vi "Determine Transmission.vi"(6 "Channel Value Change":bool, 8 "Detect?":bool[](array[boolean]), 9 "Values":dbl[](array[numeric]), 10 "Trigger VS Index":i32, 11 "Transmit Trigger":T1) -> (3 "Transmit":bool)   [LabVIEW 2015, in "Protection and Rolling Counter Addon Engine.lvlib"]
uses:
  Protection and Rolling Counter Addon Engine.lvlib
  Shared/Types/Event Trigger Type.ctl
  Shared/Protection and Rolling Counter Addon Shared.lvlib
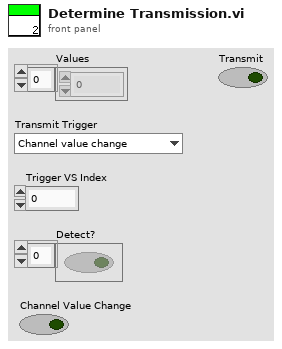
[diagram p1: front panel]
types:
  T1 = typedef "Protection and Rolling Counter Addon Shared.lvlib/Event Trigger Type.ctl" = enum16{"Channel value change", "Trigger channel (not zero)", "Channel value change or trigger channel (not zero)", "Trigger channel (any value change)", "Channel value change or trigger channel (any value change)"}
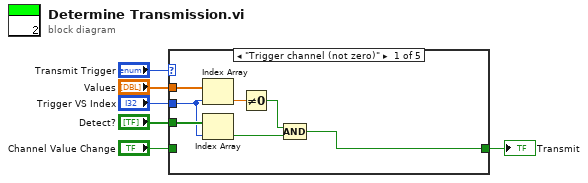
[diagram p0: block diagram]
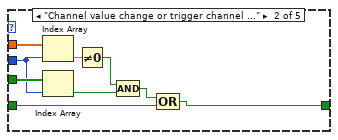
[diagram p2: hidden frame]
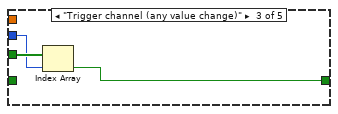
[diagram p3: hidden frame]
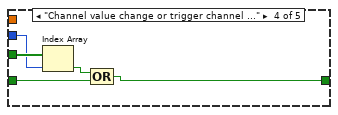
[diagram p4: hidden frame]
diagram:
  n1 = case shown="\"Trigger channel (not zero)\"" "Transmit Trigger" {
    tunnel: "Detect?" -> [w11 w22 w25 w30 _]
    tunnel: "Values" -> [w13 w21 _ _ _]
    tunnel: "Trigger VS Index" -> [w10 w20 w24 w29 _]
    tunnel: "Channel Value Change" -> [_ w15 _ w28 w31]
    tunnel: [w7 w14 w23 w26 w31] -> w6
    frame "Trigger channel (not zero)" {
      n2 = Index Array(array=w13, index=w10) -> (element=w12:dbl)
      n3 = Index Array(array=w11, index=w10) -> (element=w9:bool)
      n4 = Not Equal To 0?(x=w12) -> (x != 0?=w8:bool)
      n5 = Compound Arithmetic op=AND(w8, w9) -> (w7:bool)
    }
    frame "Channel value change or trigger channel (not zero)" {
      n6 = Index Array(array=w21, index=w20) -> (element=w19:dbl)
      n7 = Index Array(array=w22, index=w20) -> (element=w18:bool)
      n8 = Not Equal To 0?(x=w19) -> (x != 0?=w17:bool)
      n9 = Compound Arithmetic op=AND(w17, w18) -> (w16:bool)
      n10 = Compound Arithmetic op=OR(w16, w15) -> (w14:bool)
    }
    frame "Trigger channel (any value change)" {
      n11 = Index Array(array=w25, index=w24) -> (element=w23:bool)
    }
    frame "Channel value change or trigger channel (any value change)" {
      n12 = Index Array(array=w30, index=w29) -> (element=w27:bool)
      n13 = Compound Arithmetic op=OR(w27, w28) -> (w26:bool)
    }
    frame "Channel value change" {
    }
  }
  "Transmit" <- w6
